vi "MB_Master Multiple Sessions.vi"   [LabVIEW 2012]
doc: "This example opens two copies of the modbus master communication\ntester. This demonstrates how two modbus sessions can run concurrently.\n\nNote that it is possible to configure both sessions to use the same serial port.\nThis is very useful if there is more than one device on a RS-485 bus. The mobus\nmaster sessions use VISA locks to make sure that they don't interrupt eachother."
panel:
  # "This example opens two copies of the modbus master communication\ntester. This demonstrates how two modbus sessions can run concurrently.\n\nNote that it is possible to configure both sessions to use the same serial port.\nThis is very useful if there is more than one device on a RS-485 bus. The mobus\nmaster sessions use VISA locks to make sure that they don't interrupt eachother."
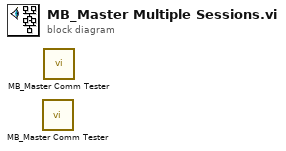
[diagram p0: block diagram]
diagram:
  n1 = call "MB_Master Comm Tester.vi"() -> ()  [unwired: 12 in]
  n2 = call "MB_Master Comm Tester.vi"() -> ()  [unwired: 12 in]
